vi "create study from images.vi"() -> ()   [LabVIEW 2023]
uses:
  study/Study.lvclass
  imaqdx-classes/imaqdx/A700/A700.lvclass
  gitlab/Multi-Sensor-Scanner/controls/General.ctl
  gitlab/thermography-acquisition/thermography-acquisition/Cam.ctl
  gitlab/thermography-acquisition/Thermography Acquisition.lvlib
  gitlab/Multi-Sensor-Scanner/controls/Series.ctl
panel:
  in  "Series List":i32(listbox)
  in  "Settings":cluster{"General":T1, "Cam":T2, "Series":T3}
  in  "Specimen":string
  in  "StudyUID":string
  in  "Path":path
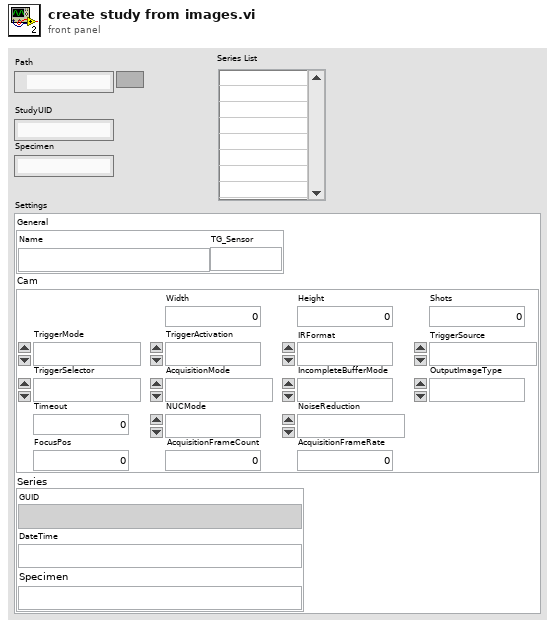
[diagram p1: front panel]
types:
  T1 = typedef "General.ctl" = cluster{"Name":string, "TG_Sensor":string}
  T2 = typedef "Thermography Acquisition.lvlib/Cam.ctl" = cluster{"Width":u32, "Height":u32, "Shots":u32, "TriggerMode":u32, "TriggerActivation":u32, "IRFormat":u32, "TriggerSource":u32, "TriggerSelector":u32, "AcquisitionMode":u32, "IncompleteBufferMode":u32, "OutputImageType":u32, "Timeout":i64, "NUCMode":u32, "NoiseReduction":u32, "FocusPos":i64, "AcquisitionFrameCount":i64, "AcquisitionFrameRate":dbl}
  T3 = typedef "Series.ctl" = cluster{"GUID":string, "DateTime":string, "Specimen":string}
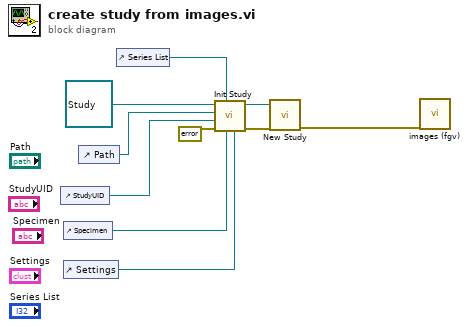
[diagram p0: block diagram]
diagram:
  n1 = control-ref of="StudyUID"() -> (w8:refnum<vi>)
  n2 = control-ref of="Specimen"() -> (w6:refnum<vi>)
  n3 = control-ref of="Settings"() -> (w5:refnum<vi>)
  n4 = control-ref of="Path"() -> (w9:refnum<vi>)
  n5 = control-ref of="Series List"() -> (w2:refnum<vi>)
  n6 = call "Init Study.vi"("Applied Settings Cluster Ref"=w5, "Specimen Ref"=w6, "Series List Ref"=w2, "error in (no error)"=errorcluster {"status"=FALSE, "code"=0, "source"=""}, "Study UID Ref"=w8, "File Refnum"=w9, "Study in"=refnum<class "Study.lvclass"> refnum) -> ("error out"=w4:errorcluster, "Study out"=w7:refnum<class "Study.lvclass">)  [unwired: 3 in]
  n7 = call "New Study.vi"("error in (no error)"=w4, "Study in"=w7) -> ("error out"=w1:errorcluster)  [unwired: 8 in, 1 out]
  n8 = call "images (fgv).vi"("Error in"=w1) -> ()  [unwired: 7 in, 4 out]
